vi "libssh2_userauth_publickey.vi"(7 "sign":refnum<vi>, 8 "error in (no error)":errorcluster, 9 "public key data":u8[](array[numeric]), 10 "username":string, 11 "session":T1) -> (0 "error out":errorcluster)   [LabVIEW 2017, in "libssh2.lvlib"]
doc: "Authenticate a session using a public key and a custom signing function.\n\nThis function utilizes the lvssh2 extension library. You can disable the extension library by defining the LVSSH2_NO_EXTENSIONS conditional disable symbol with the value 'True' in the project properties. When the extension library is disabled, this function turns into a no-op."
uses:
  libssh2.lvlib
  Session Refnum.ctl
  lvssh2_userauth_publickey_sign_function_input_args_64.ctl
  Not A Session.vi
  Global Settings.vi
  lvssh2_userauth_publickey_sign_function_handler_64.vi
  Read Session Refnum.vi
  <vilib>/Utility/semaphor.llb/Acquire Semaphore.vi
  <vilib>/Utility/semaphor.llb/Release Semaphore.vi
  lvssh2_userauth_publickey_sign_function_handler_32.vi
  lvssh2_userauth_publickey_sign_function_input_args_32.ctl
  lvssh2_extensions_64.dll
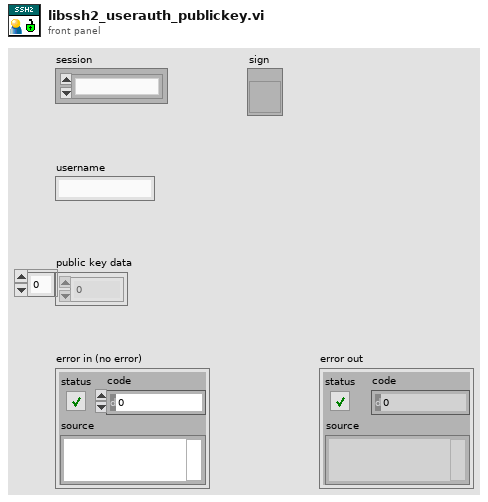
[diagram p1: front panel]
types:
  T1 = typedef "libssh2.lvlib/Session Refnum.ctl" = refnum<k1>
  T2 = typedef "libssh2.lvlib/lvssh2_userauth_publickey_sign_function_input_args_64.ctl" = cluster{"data":u8[], "*signature":u64, "completion":u64}
  T3 = typedef "libssh2.lvlib/lvssh2_userauth_publickey_sign_function_input_args_32.ctl" = cluster{"data":u8[], "*signature":u32, "completion":u32}
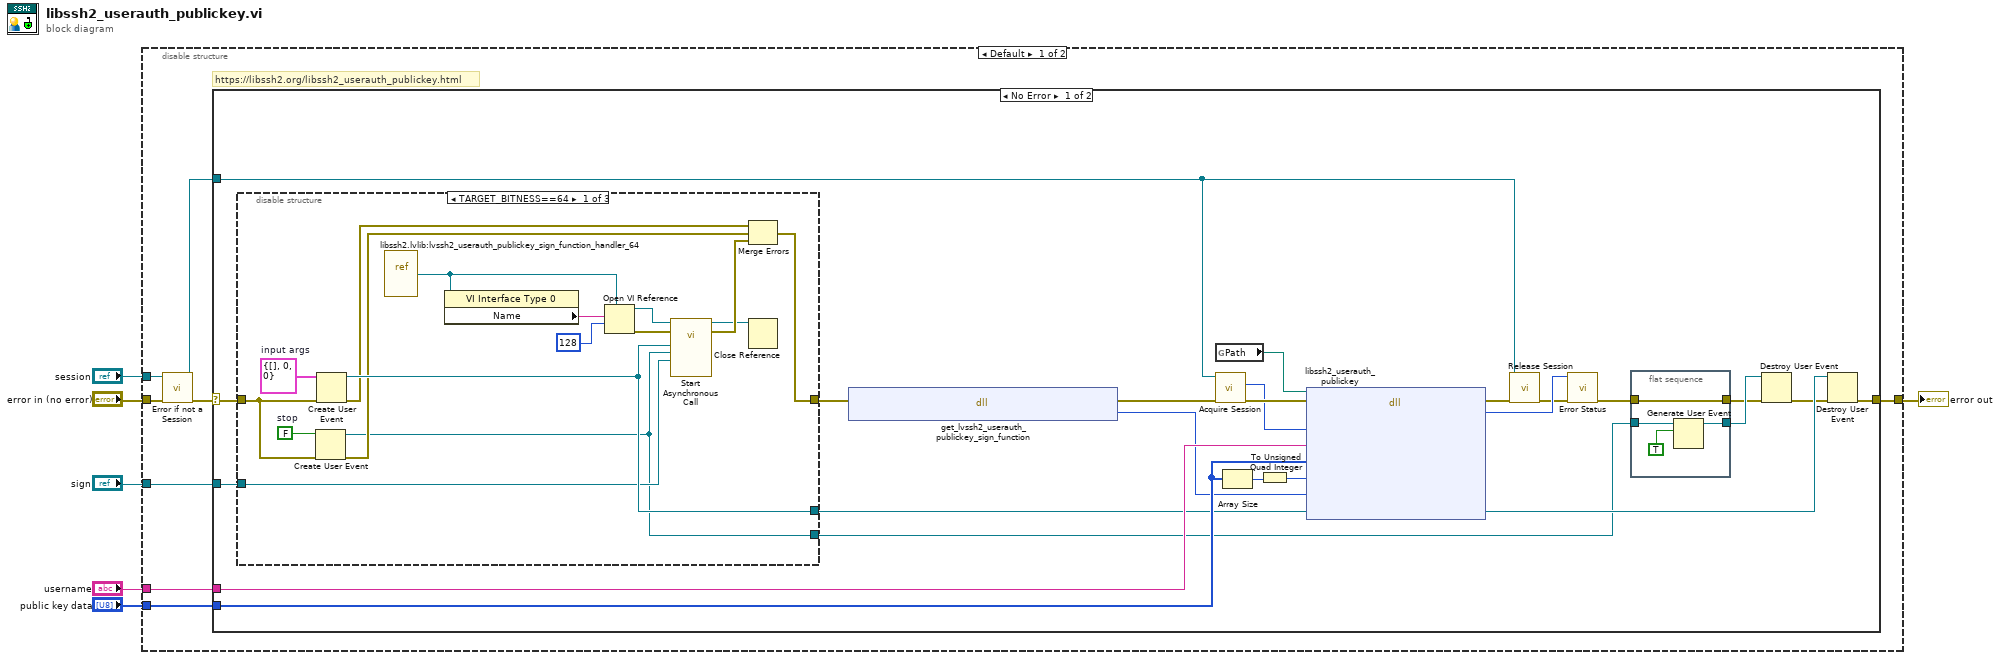
[diagram p0: block diagram]
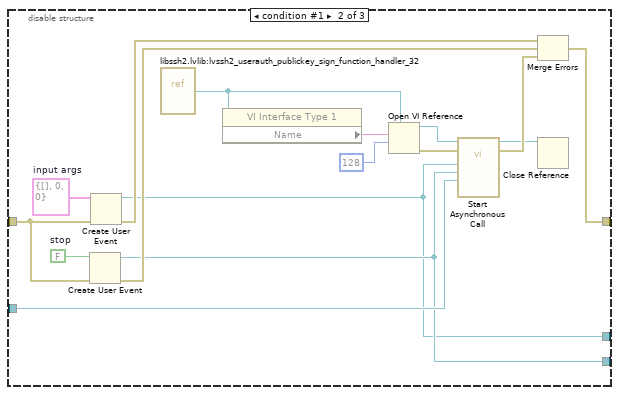
[diagram p2: hidden frame]
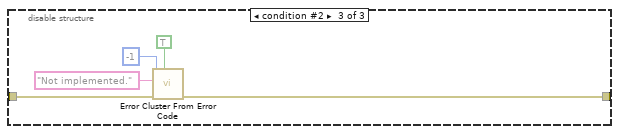
[diagram p3: hidden frame]
diagram:
  n1 = disable-structure shown="Default" {
    disable-tunnel: "username" -> [w14 _]
    disable-tunnel: [w13 w81] -> w5
    disable-tunnel: "error in (no error)" -> [w12 w81]
    disable-tunnel: "session" -> [w10 _]
    disable-tunnel: "public key data" -> [w8 _]
    disable-tunnel: "sign" -> [w7 _]
    frame condition #0 (active) {
      # "https://libssh2.org/libssh2_userauth_publickey.html"
      n2 = call "Error if not a Session.vi"("error in (no error)"=w12, "session"=w10) -> ("error out"=w11:errorcluster, "session out"=w9:T1)  [unwired: 8 in]
      n3 = case shown="No Error" w11 {
        selector: w11 -> [w25 w80]
        tunnel: w14 -> [w38 _]
        tunnel: [w24 w80] -> w13
        tunnel: w9 -> [w20 _]
        tunnel: w8 -> [w31 _]
        tunnel: w7 -> [w27 _]
        frame No Error {
          n4 = disable-structure shown="TARGET_BITNESS==64" {
            disable-tunnel: w27 -> [w50 w69 _]
            disable-tunnel: [w45 w64 w78] -> w26
            disable-tunnel: w25 -> [w49 w68 w79]
            disable-tunnel: [w52 w60 _] -> w23
            disable-tunnel: [w44 w63 _] -> w17
            frame condition #0 (active) {
              w51 = FALSE  # stop
              w58 = T2 {"data"=[], "*signature"=0, "completion"=0}  # input args
              n5 = Create User Event(user event datatype=w51, error in=w49) -> (user event=w44:refnum<user-event>, error out=w47:errorcluster)
              n6 = Create User Event(user event datatype=w58, error in=w49) -> (user event=w52:refnum<user-event>, error out=w48:errorcluster)
              n7 = vi-ref "libssh2.lvlib:lvssh2_userauth_publickey_sign_function_handler_64.vi"() -> (w53:refnum<vi>)
              n8 = property class="VI Interface Type 0"(reference=w53) -> ("Name"=w57:string)  [unwired: 1 in, 2 out]
              n9 = Open VI Reference(type specifier VI Refnum (for type only)=w53, vi path=w57, options=128) -> (vi reference=w54:refnum<vi>, error out=w55:errorcluster)  [unwired: 3 in]
              n10 = call-by-ref "Start Asynchronous Call"(reference=w54, error in=w55, "lvssh2_userauth_publickey_sign_function"=w50, "Stop Event Ref"=w44, "User Event Ref"=w52) -> (reference out=w43:refnum<vi>, error out=w46:errorcluster)  [unwired: 9 in]
              n11 = Merge Errors(w48, w47, w46) -> (w45:errorcluster)
              n12 = Close Reference(reference=w43) -> ()  [unwired: 1 in, 1 out]
            }
            frame condition #1 {
              w62 = T3 {"data"=[], "*signature"=0, "completion"=0}  # input args
              w70 = FALSE  # stop
              n13 = Create User Event(user event datatype=w70, error in=w68) -> (user event=w63:refnum<user-event>, error out=w66:errorcluster)
              n14 = Create User Event(user event datatype=w62, error in=w68) -> (user event=w60:refnum<user-event>, error out=w67:errorcluster)
              n15 = vi-ref "libssh2.lvlib:lvssh2_userauth_publickey_sign_function_handler_32.vi"() -> (w61:refnum<vi>)
              n16 = property class="VI Interface Type 1"(reference=w61) -> ("Name"=w74:string)  [unwired: 1 in, 2 out]
              n17 = Open VI Reference(type specifier VI Refnum (for type only)=w61, vi path=w74, options=128) -> (vi reference=w71:refnum<vi>, error out=w72:errorcluster)  [unwired: 3 in]
              n18 = call-by-ref "Start Asynchronous Call"(reference=w71, error in=w72, "lvssh2_userauth_publickey_sign_function"=w69, "Stop Event Ref"=w63, "User Event Ref"=w60) -> (reference out=w59:refnum<vi>, error out=w65:errorcluster)  [unwired: 9 in]
              n19 = Merge Errors(w67, w66, w65) -> (w64:errorcluster)
              n20 = Close Reference(reference=w59) -> ()  [unwired: 1 in, 1 out]
            }
            frame condition #2 {
              n21 = call <vilib>:"Error Cluster From Error Code.vi"("show call chain? (False)"=TRUE, "error in (no error)"=w79, "error message (\"\")"="Not implemented." ("error message (\"\")"), "error code (0)"=-1) -> ("error out"=w78:errorcluster)  [unwired: 5 in]
            }
          }
          n22 = dll-call lib="C:/Users/pasca/Projects/Home/lvssh2/libssh2/lvssh2_extensions**.*" fn="get_lvssh2_userauth_publickey_sign_function"(error in=w26) -> (error out=w29:errorcluster, "return type"=w28:u64)  [unwired: 2 in, 1 out]
          n23 = global read "Global Settings.vi" "Path"() -> (w34:path)
          n24 = call "Acquire Session.vi"("error in (no error)"=w29, "session"=w20) -> ("error out"=w36:errorcluster, "LIBSSH2_SESSION*"=w35:u64)  [unwired: 7 in, 1 out]
          n25 = Array Size(array=w31) -> (size(s)=w32:i32)
          n26 = To Unsigned Quad Integer(1:w32) -> (0:w30:u64)
          n27 = dll-call lib="?" fn="libssh2_userauth_publickey"(path in=w34, error in=w36, "session"=w35, "username"=w38, "pubkeydata"=w31, "pubkeydata_len"=w30, "sign_callback"=w28, "abstract"=w23) -> (error out=w37:errorcluster, "return value"=w33:i32, "abstract"=w22:refnum<user-event>)  [unwired: 6 in, 1 out]
          n28 = call "Release Session.vi"("error in (no error)"=w37, "session"=w20) -> ("error out"=w21:errorcluster)  [unwired: 9 in]
          n29 = call "Error Status.vi"("error in (no error)"=w21, "return value"=w33) -> ("error out"=w15:errorcluster)  [unwired: 8 in, 1 out]
          n30 = flat-sequence {
            tunnel: [w42] -> w18
            tunnel: w17 -> [w40]
            tunnel: [w39] -> w16
            tunnel: w15 -> [w39]
            frame #0 {
              n31 = Generate User Event(user event=w40, event data cluster=TRUE ("event data")) -> (user event out=w42:refnum<user-event>)  [unwired: 2 in, 1 out]
            }
          }
          n32 = Destroy User Event(user event=w18, error in=w16) -> (error out=w19:errorcluster)
          n33 = Destroy User Event(user event=w22, error in=w19) -> (error out=w24:errorcluster)
        }
        frame Error {
        }
      }
    }
    frame condition #1 {
    }
  }
  "error out" <- w5
